vi "Acquire_PID_Tests_steps_ctrOnOffAlt.vi"() -> ()   [LabVIEW 2016]
uses:
  Globals/PressuresGlobal.vi
panel:
  in  "Control Valve":enum16{"1", "2", "3", "4", "5", "6", "7", "8"}(ring)=enum."7"
  out "Exp Time":dbl
  in  "Time_Stable(s)":dbl=30.0
  in  "Wait For Microscope?":bool=TRUE
  in  "stop2":bool
  in  "Flow Path":path=path "E:/maggot images/Jacob/20171121/stepTest20units_run101.mat"
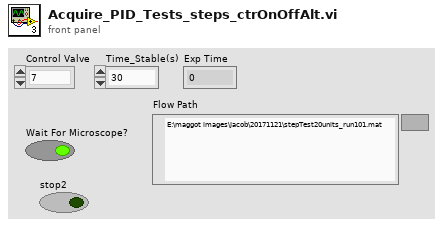
[diagram p1: front panel]
types:
  T1 = cluster{"relative seconds":dbl, "Pressures":dbl[], "F1 PID gains":dbl[], "FTot PID gains":dbl[], "PID On?":i16, "flow setpoints":dbl[]}
  T2 = cluster{"Time":dbl, "All Flow-Rates":dbl[], "Flow 2 Filter Time":dbl, "Flow 1 Filter Time":dbl}
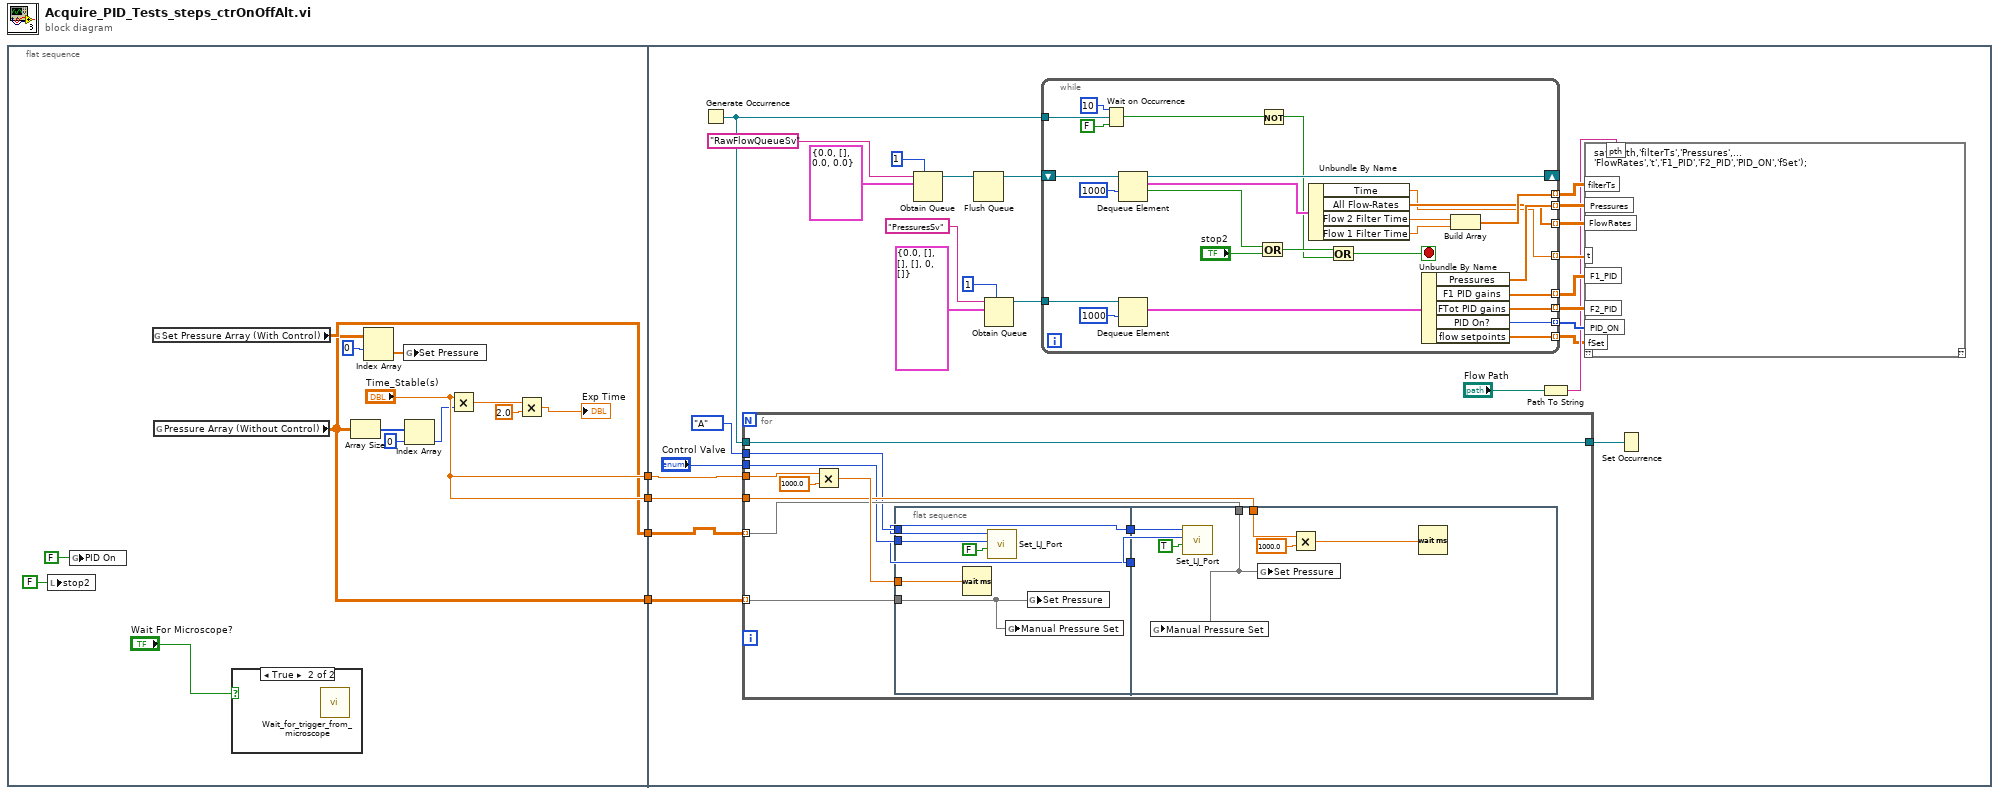
[diagram p0: block diagram]
diagram:
  n1 = flat-sequence {
    tunnel: ["Time_Stable(s)"] -> w4
    tunnel: ["Time_Stable(s)"] -> w3
    tunnel: [w10] -> w2
    tunnel: [w13] -> w1
    tunnel: w4 -> [w26]
    tunnel: w3 -> [w23]
    tunnel: w2 -> [w20]
    tunnel: w1 -> [w19]
    frame #0 {
      n2 = local write "stop2"(FALSE ("stop2")) -> ()
      n3 = global write "PressuresGlobal.vi" "PID On"(FALSE ("PID On")) -> ()
      n4 = global read "PressuresGlobal.vi" "Set Pressure Array (With Control)"() -> (w13:dbl[][])
      n5 = global read "PressuresGlobal.vi" "Pressure Array (Without Control)"() -> (w10:dbl[][])
      n6 = case shown="True" "Wait For Microscope?" {
        frame False {
        }
        frame True {
          n7 = call "Wait_for_trigger_from_microscope.vi"() -> ()  [unwired: 12 in]
        }
      }
      n8 = Array Size(array=w10) -> (size(s)=w9:i32[])
      n9 = Index Array(array=w10, index (row)=0) -> (element=w11:dbl[])  [unwired: 1 in]
      n10 = global write "PressuresGlobal.vi" "Set Pressure"(w11) -> ()
      n11 = Index Array(array=w9, index=0) -> (element=w8:i32)
      n12 = Multiply(x="Time_Stable(s)", y=w8) -> (x*y=w16:dbl)
      n13 = Multiply(x=w16, y=2.0) -> (x*y=→"Exp Time":dbl)
    }
    frame #1 {
      n14 = Generate Occurrence() -> (w25:refnum<k4>)
      n15 = for {
        tunnel: w26 -> [w54]
        tunnel: w25 -> [w53]
        tunnel: [w53] -> w24
        tunnel: w23 -> [w52]
        tunnel: w20 -> [w50] mode=indexing
        tunnel: w19 -> [w51] mode=indexing
        tunnel: "Control Valve" -> [w49]
        tunnel: enum16{"A", "B", "C"}."A" ("Flowboard") -> [w48]
        n16 = Multiply(x=w52, y=1000.0) -> (x*y=w55:dbl)
        n17 = flat-sequence {
          tunnel: w55 -> [w61]
          tunnel: w50 -> [w57]
          tunnel: w49 -> [w58]
          tunnel: w48 -> [w59]
          tunnel: [w59] -> w47
          tunnel: [w58] -> w46
          tunnel: w54 -> [w67]
          tunnel: w51 -> [w62]
          tunnel: w47 -> [w65]
          tunnel: w46 -> [w64]
          frame #0 {
            n18 = Wait (ms)(milliseconds to wait=w61) -> ()  [unwired: 1 out]
            n19 = call "Set_LJ_Port.vi"("State"=FALSE, "Channel"=w58, "Flowboard"=w59) -> ()  [unwired: 8 in, 1 out]
            n20 = global write "PressuresGlobal.vi" "Manual Pressure Set"(w57) -> ()
            n21 = global write "PressuresGlobal.vi" "Set Pressure"(w57) -> ()
          }
          frame #1 {
            n22 = global write "PressuresGlobal.vi" "Manual Pressure Set"(w62) -> ()
            n23 = call "Set_LJ_Port.vi"("State"=TRUE, "Channel"=w64, "Flowboard"=w65) -> ()  [unwired: 8 in, 1 out]
            n24 = global write "PressuresGlobal.vi" "Set Pressure"(w62) -> ()
            n25 = Multiply(x=w67, y=1000.0) -> (x*y=w68:dbl)
            n26 = Wait (ms)(milliseconds to wait=w68) -> ()  [unwired: 1 out]
          }
        }
      }
      n27 = Obtain Queue(max queue size (-1, unlimited)=1, name (unnamed)="RawFlowQueueSv", element data type=T2 {"Time"=0.0, "All Flow-Rates"=[], "Flow 2 Filter Time"=0.0, "Flow 1 Filter Time"=0.0} ("output cluster")) -> (queue out=w44:refnum<queue>)  [unwired: 2 in, 2 out]
      n28 = Flush Queue(queue=w44) -> (queue out=w43:refnum<queue>)  [unwired: 1 in, 2 out]
      n29 = Obtain Queue(max queue size (-1, unlimited)=1, name (unnamed)="PressuresSv", element data type=T1 {"relative seconds"=0.0, "Pressures"=[], "F1 PID gains"=[], "FTot PID gains"=[], "PID On?"=0, "flow setpoints"=[]} ("output cluster")) -> (queue out=w39:refnum<queue>)  [unwired: 2 in, 2 out]
      n30 = while {
        shift-right: [w91] -> _
        shift-left: w43 -> [w94]
        tunnel: w39 -> [w88]
        tunnel: [w83] -> w30 mode=indexing
        tunnel: [w82] -> w31 mode=indexing
        tunnel: [w81] -> w32 mode=indexing
        tunnel: [w80] -> w34 mode=indexing
        tunnel: [w79] -> w36 mode=indexing
        tunnel: [w78] -> w35 mode=indexing
        tunnel: [w77] -> w33 mode=indexing
        tunnel: [w76] -> w27 mode=indexing
        tunnel: w25 -> [w75]
        stop <- w70 stop-if-true
        n31 = Wait on Occurrence(1:FALSE ("ignore previous (T)"), 2:w75, 3:10 ("ms timeout (-1)")) -> (0:w72:bool)
        n32 = Dequeue Element(queue=w94, timeout in ms (-1)=1000) -> (queue out=w91:refnum<queue>, element=w87:T2, timed out?=w92:bool)  [unwired: 1 in, 1 out]
        n33 = Dequeue Element(queue=w88, timeout in ms (-1)=1000) -> (element=w84:T1)  [unwired: 1 in, 3 out]
        n34 = Or(x=w92, y="stop2") -> (x .or. y?=w71:bool)
        n35 = Not(x=w72) -> (.not. x?=w69:bool)
        n36 = Unbundle By Name(w87) -> ("Time"=w77:dbl, "All Flow-Rates"=w78:dbl[], "Flow 2 Filter Time"=w86:dbl, "Flow 1 Filter Time"=w85:dbl)
        n37 = Or(x=w71, y=w69) -> (x .or. y?=w70:bool)
        n38 = Unbundle By Name(w84) -> ("Pressures"=w80:dbl[], "F1 PID gains"=w81:dbl[], "FTot PID gains"=w82:dbl[], "PID On?"=w83:i16, "flow setpoints"=w76:dbl[])
        n39 = Build Array(w86, w85) -> (w79:dbl[])
      }
      n40 = Path To String(path="Flow Path") -> (string=w29:string)
      n41 = script code="save(pth,'filterTs','Pressures',...\n'FlowRates','t','F1_PID','F2_PID','PID_ON','fSet');"("pth"=w29, "t"=w33, "F1_PID"=w32, "F2_PID"=w31, "PID_ON"=w30, "Pressures"=w34, "FlowRates"=w35, "filterTs"=w36, "fSet"=w27) -> ()  [unwired: 1 in, 1 out]
      n42 = Set Occurrence(w24) -> ()
    }
  }
